vi "load_from_db.vi"() -> (0 "db_name":string, 1 "Result Set":string[][](table) caption="Result Set (from first statement with results)")   [LabVIEW 2013]
uses:
  <vilib>/drjdpowell/SQLite Library/SQL Connection/Connection.lvclass
  <vilib>/drjdpowell/SQLite Library/SQL Connection/Open (path).vi
  <vilib>/drjdpowell/SQLite Library/SQL Connection/Open (string).vi
  <vilib>/AdvancedString/Path To Command Line String.vi
panel:
  in  "DatabaseList":string(combo)
  in  "Cancel":bool
  in  "Load":bool
  # "Wybierz bazê danych do wczytania:"
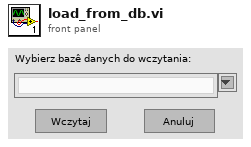
[diagram p1: front panel]
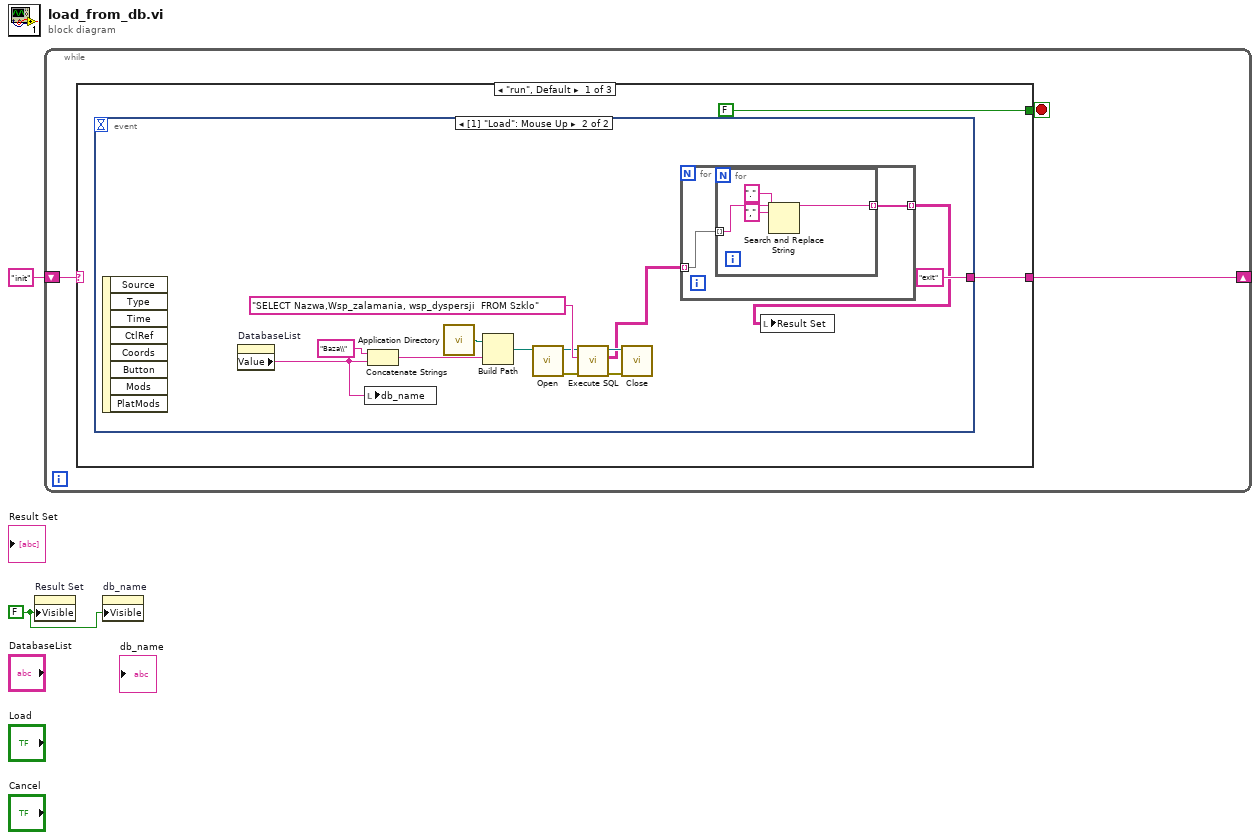
[diagram p0: block diagram]
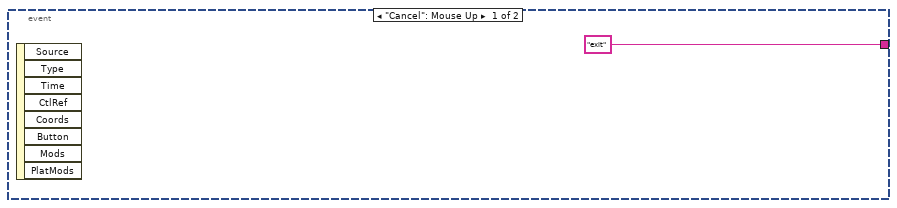
[diagram p2: hidden frame]
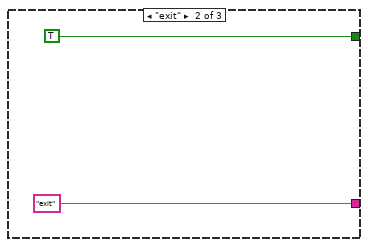
[diagram p3: hidden frame]
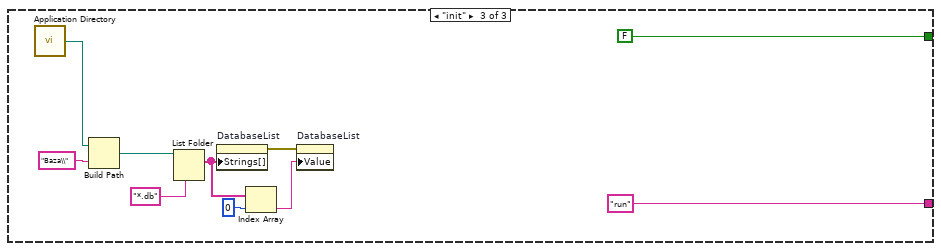
[diagram p4: hidden frame]
diagram:
  w1 = FALSE ("Visible")
  n1 = property on="Result Set" class="Tbl (strict)"("Visible"=w1) -> ()  [unwired: 2 in, 2 out]
  n2 = while {
    shift-right: [w4] -> _
    shift-left: "init" -> [w5]
    stop <- w3 stop-if-true
    n3 = case shown="\"run\", Default" w5 {
      tunnel: [w7 "exit" "run"] -> w4
      tunnel: [FALSE TRUE FALSE] -> w3
      frame "run", Default {
        n4 = event shown="[1] \"Load\": Mouse Up" {
          selector: _ -> [_ _]
          dyn-events: _ -> [_ _]
          timeout: _ -> [_ _]
          tunnel: ["exit" "exit"] -> w7
          event "Cancel": Mouse Up {
            n5 = event-data() -> ()  [unwired: 1 in, 8 out]
          }
          event "Load": Mouse Up {
            n6 = event-data() -> ()  [unwired: 1 in, 8 out]
            n7 = property on="DatabaseList" class="CmbBox"() -> ("Value"=w9:string)  [unwired: 2 in, 2 out]
            n8 = local write "db_name"(w9) -> ()
            n9 = Concatenate Strings("Baza\\" ("db file"), w9) -> (w12:string)
            n10 = call <vilib>:"Application Directory.vi"() -> ("Application Directory"=w15:path)
            n11 = Build Path(base path=w15, name or relative path=w12) -> (appended path=w19:path)
            n12 = call-poly <vilib>:"Open.vi"("db file"=w19) -> ("error out"=w17:errorcluster, "SQLite Connection out"=w18:refnum<class "Connection.lvclass">)  [unwired: 9 in]
            n13 = call <vilib>:"Execute SQL.vi"("error in (no error)"=w17, "SQL"="SELECT Nazwa,Wsp_zalamania, wsp_dyspersji  FROM Szklo" ("SELECT  statement"), "SQLite Connection in"=w18) -> ("error out"=w14:errorcluster, "Result Set"=w11:string[][], "SQLite Connection out"=w13:refnum<class "Connection.lvclass">)  [unwired: 5 in, 1 out]
            n14 = call-dynamic "Close.vi"("error in (no error)"=w14, "SQLite Connection in"=w13) -> ()  [unwired: 9 in, 1 out]
            n15 = for {
              tunnel: w11 -> [w23] mode=indexing
              tunnel: [w22] -> w10 mode=indexing
              n16 = for {
                tunnel: w23 -> [w27] mode=indexing
                tunnel: [w24] -> w22 mode=indexing
                n17 = Search and Replace String(input string=w27, search string=",", replace string="." ("replace string (\"\")")) -> (result string=w24:string)  [unwired: 5 in, 3 out]
              }
            }
            n18 = local write "Result Set"(w10) -> ()
          }
        }
      }
      frame "exit" {
      }
      frame "init" {
        n19 = call <vilib>:"Application Directory.vi"() -> ("Application Directory"=w39:path)
        n20 = Build Path(base path=w39, name or relative path="Baza\\") -> (appended path=w37:path)
        n21 = List Folder(path=w37, pattern="*.db") -> (filenames=w34:string[])  [unwired: 2 in, 3 out]
        n22 = property on="DatabaseList" class="CmbBox"("Strings[]"=w34) -> (error out=w35:errorcluster)  [unwired: 2 in, 1 out]
        n23 = Index Array(array=w34, index=0) -> (element=w32:string)
        n24 = property on="DatabaseList" class="CmbBox"(error in=w35, "Value"=w32) -> ()  [unwired: 1 in, 2 out]
      }
    }
  }
  n25 = property on="db_name" class="Str"("Visible"=w1) -> ()  [unwired: 2 in, 2 out]
